vi "Create Image Queues.vi"(8 "error in (no error)":errorcluster, 9 "Buffers":i32=2 min=1 max=2, 10 "Chunk Size":u32=1048576, 11 "Image Size":u32=3456032) -> (0 "error out":errorcluster, 3 "Image Transfer Parameters":T1={"Image Queue"=refnum, "Return Queue"=refnum, "Chunk Size"=1048576, "Frame Fragments"=4, "DVRs"=[]})   [LabVIEW 2021, in "DecodetoImage.lvlib"]
uses:
  DecodetoImage.lvlib
  Typedef/Image Transfer Parameters.ctl
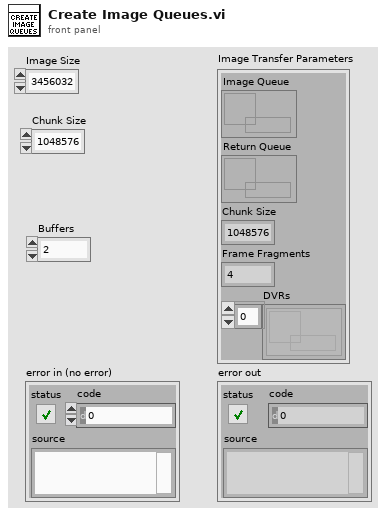
[diagram p1: front panel]
types:
  T1 = typedef "DecodetoImage.lvlib/Image Transfer Parameters.ctl" = cluster{"Image Queue":refnum<queue>, "Return Queue":refnum<queue>, "Chunk Size":u32, "Frame Fragments":u32, "DVRs":refnum<data-value>[]}
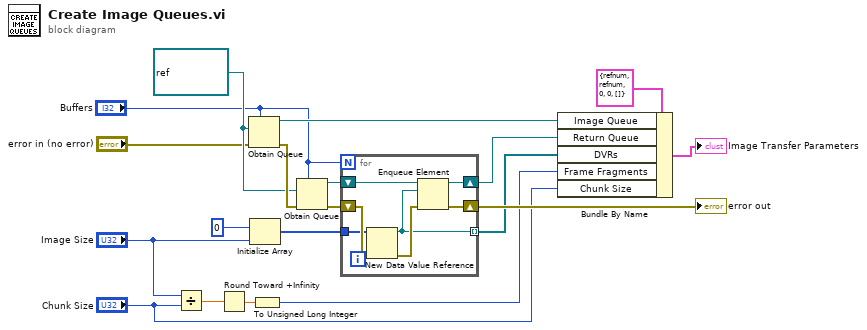
[diagram p0: block diagram]
diagram:
  w11 = refnum<data-value> refnum ("data value reference")
  n1 = Divide(x="Image Size", y="Chunk Size") -> (x/y=w18:dbl)
  n2 = Round Toward +Infinity(x=w18) -> (ceil(x): smallest int >= x=w19:dbl)
  n3 = Obtain Queue(max queue size (-1, unlimited)="Buffers", element data type=w11, error in (no error)="error in (no error)") -> (queue out=w7:refnum<queue>, error out=w15:errorcluster)  [unwired: 2 in, 1 out]
  n4 = Initialize Array(u8 0, "Image Size") -> (w13:u8[])
  n5 = To Unsigned Long Integer(number=w19) -> (unsigned 32bit integer=w5:u32)
  n6 = Obtain Queue(max queue size (-1, unlimited)="Buffers", element data type=w11, error in (no error)=w15) -> (queue out=w12:refnum<queue>, error out=w14:errorcluster)  [unwired: 2 in, 1 out]
  n7 = for {
    N: "Buffers" -> [_]
    tunnel: w13 -> [w23]
    shift-right: [w26] -> w16
    shift-left: w14 -> [w24]
    shift-right: [w21] -> w6
    shift-left: w12 -> [w22]
    tunnel: [w20] -> w1 mode=indexing
    n8 = New Data Value Reference(data value=w23, error in=w24) -> (data value reference=w20:refnum<data-value>, error out=w25:errorcluster)
    n9 = Enqueue Element(queue=w22, element=w20, error in (no error)=w25) -> (queue out=w21:refnum<queue>, error out=w26:errorcluster)  [unwired: 1 in, 1 out]
  }
  "error out" <- w16
  n10 = Bundle By Name(cluster=T1 {"Image Queue"=refnum, "Return Queue"=refnum, "Chunk Size"=0, "Frame Fragments"=0, "DVRs"=[]} ("Image Transfer Parameters 2"), "Image Queue"=w7, "Return Queue"=w6, "DVRs"=w1, "Frame Fragments"=w5, "Chunk Size"="Chunk Size") -> (→"Image Transfer Parameters":T1)
